vi "maze_v2.vi"   [LabVIEW 2012]
uses:
  <vilib>/NXT/Subs/MotorOutput.ctl
  <vilib>/NXT/Block Support/NXT_InputPort.ctl
  <vilib>/NXT/Dual Mode Library/Motors/MotorOn.vi
  <vilib>/NXT/Dual Mode Library/Motors/MotorReverse.vi
  <vilib>/NXT/Dual Mode Library/Motors/MotorBrake.vi
  <vilib>/NXT/Dual Mode Library/Display/clearDisplay.vi
  <vilib>/NXT/Dual Mode Library/Display/drawText.vi
  <vilib>/NXT/Dual Mode Library/Waits/Wait_Num(msec).vi
  <vilib>/NXT/Dual Mode Library/Display/drawLine.vi
  <vilib>/NXT/Dual Mode Library/Waits/Wait_Num.vi
  <vilib>/NXT/Dual Mode Library/Display/drawNumber.vi
types:
  T1 = typedef "MotorOutput.ctl" = u8
  T2 = typedef "LVHSConnector.ctl" = cluster{"Hardware":string, "Flattened String":string}
  T3 = typedef "NXT_InputPort.ctl" = u8
  T4 = cluster{"x":i32, "Start X":i16, "x":i32, "Start X":i16}
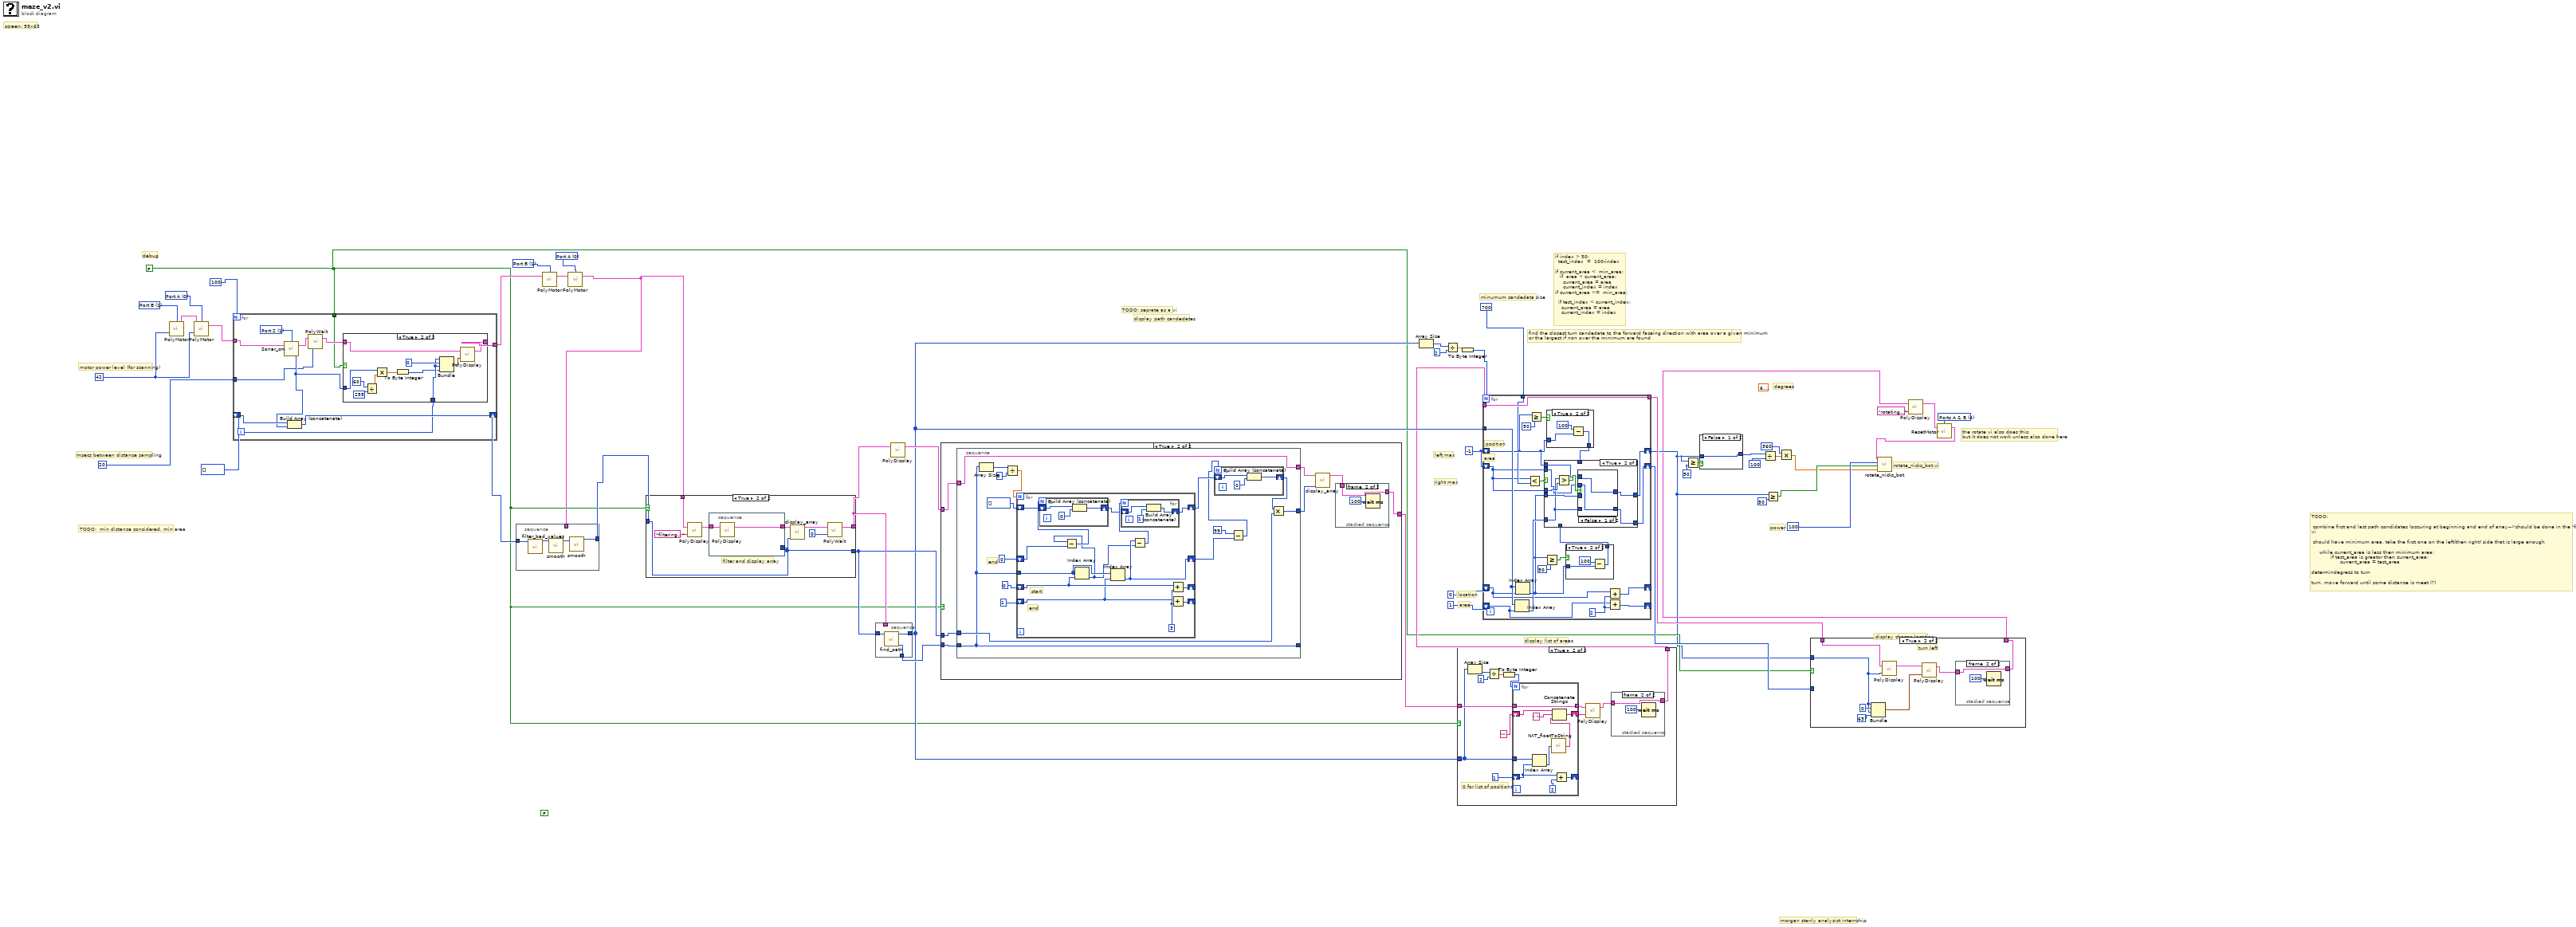
[diagram p0: block diagram]
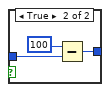
[diagram p2: hidden frame]
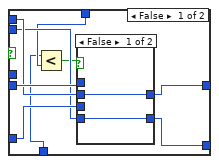
[diagram p8: hidden frame]
diagram:
  w5 = T1 4 items=["Port A"=0, "Port B"=1, "Port C"=2, "Ports A & B"=4, "Ports A & C"=5, "Ports B & C"=6, "All Ports"=3] ("Port (All Ports)")
  (unwired) 6.283185307179586 ("Pi Multiplied By 2")
  w21 = i16 -1 ("Start X")
  w38 = T1 0 items=["Port A"=0, "Port B"=1, "Port C"=2, "Ports A & B"=4, "Ports A & C"=5, "Ports B & C"=6, "as"=3] ("Output Port (All Ports)")
  w40 = T1 1 items=["Port A"=0, "Port B"=1, "Port C"=2, "Ports A & B"=4, "Ports A & C"=5, "Ports B & C"=6, "as"=3] ("Output Port (All Ports)")
  (unwired) FALSE
  w19 = FALSE
  w45 = 42 ("Power (75)")
  w47 = T1 0 items=["Port A"=0, "Port B"=1, "Port C"=2, "Ports A & B"=4, "Ports A & C"=5, "Ports B & C"=6, "as"=3] ("Output Port (All Ports)")
  w49 = T1 1 items=["Port A"=0, "Port B"=1, "Port C"=2, "Ports A & B"=4, "Ports A & C"=5, "Ports B & C"=6, "as"=3] ("Output Port (All Ports)")
  # "rotate_nicks_bot.vi"
  # "the rotate vi also does this,\nbut it does not work unless also done here"
  # "power"
  # "degrees"
  # "display chosen location"
  # "display list of areas"
  # "if index > 50;\n  test_index  =  100-index\n\nif current_area <  min_area:\n   if  area > current_area:\n     current_area = area\n     current_index = index\nif current_area >=  min_area:\n\n  if test_index < current_index:\n    current_area = area\n    current_index = index"
  # "morgan stanly analysist internship"
  # "minumum candedata size"
  # "find the closest turn candedate to the forward faceing direction with area over a given minimum\nor the largest if non over the minimum are found"
  # "TODO:  min distance considered, min area"
  # "msecs between distance sampling"
  # "motor power level (for scanning)"
  # "TODO: seprate as a vi"
  # "TODO:\n\n combine first and last path condidates (occuring at beginning and end of array-->should be done in the 'find paths' vi\n            \n should have minimum area, take the first one on the left(then right) side that is large enough\n\n     while current_area is less then minimum area:\n            if test_area is greator then current_area:\n                  current_area = test_area\n\ndetermindegress to turn\n\nturn, move forward until some distance is meet (?)"
  # "right max"
  # "left max"
  # "display path candedates"
  # "area"
  # "location"
  # "debug"
  # "screen: 99x63"
  n1 = call-poly <vilib>:"PolyMotor.vi"("Power (75)"=w45, "Output Port (All Ports)"=w49) -> ("NXT"=w48:T2)  [unwired: 2 in]
  n2 = call-poly <vilib>:"PolyMotor.vi"("Power (75)"=w45, "NXT"=w48, "Output Port (All Ports)"=w47) -> ("NXT"=w46:T2)  [unwired: 1 in]
  n3 = for {
    N: 100 -> [_]
    shift-right: [w57] -> w42
    shift-left: i16[] [] -> [w58]
    tunnel: w46 -> [w60]
    tunnel: [w54] -> w39
    tunnel: w19 -> [w53]
    tunnel: 20 -> [w50]
    i -> [w51]
    w59 = T3 1 items=["Port 1", "Port 2", "Port 3", "Port 4"] ("Port (Port 4)")
    n4 = call <vilib>:"Sonar_cm.vi"("NXT"=w60, "Port (Port 4)"=w59) -> ("Distance (cm)"=w52:i16, "NXT"=w56:T2)  [unwired: 1 in]
    n5 = Build Array (concatenate)(w58, w52) -> (w57:i16[])
    n6 = call-poly <vilib>:"PolyWait.vi"("Time (100 msec)"=w50, "NXT"=w56) -> ("NXT"=w55:T2)  [unwired: 2 in]
    n7 = case shown="True" w53 {
      tunnel: w55 -> [w61 w69]
      tunnel: [w61 w70] -> w54
      tunnel: w52 -> [_ w68]
      tunnel: w51 -> [_ w63]
      frame False {
      }
      frame True {
        n8 = Divide(x=i16 60 ("Start X"), y=i16 255 ("Start X")) -> (x/y=w66:dbl)
        n9 = Multiply(x=w68, y=w66) -> (x*y=w71:dbl)
        n10 = To Byte Integer(number=w71) -> (8bit integer=w62:i8)
        n11 = Bundle(w63, "Start X"=i16 0, w63, w62) -> (w64:cluster{i32, "Start X":i16, i32, i8})  [unwired: 1 in]
        n12 = call-poly <vilib>:"PolyDisplay.vi"("Line Parameters"=w64, "NXT"=w69) -> ("NXT"=w70:T2)  [unwired: 2 in]
      }
    }
  }
  n13 = call-poly <vilib>:"PolyMotor.vi"("NXT"=w39, "Port (All Ports)"=w40) -> ("NXT"=w41:T2)  [unwired: 2 in]
  n14 = call-poly <vilib>:"PolyMotor.vi"("NXT"=w41, "Port (All Ports)"=w38) -> ("NXT"=w1:T2)  [unwired: 2 in]
  n15 = stacked-sequence {
    tunnel: w42 -> [w74]
    tunnel: [w73] -> w37
    tunnel: w1 -> [_]
    frame #0 {
      n16 = call "filter_bad_values.vi"("Array 3"=w74) -> ("Array 4"=w75:i32[])  [unwired: 10 in]
      n17 = call "smooth.vi"("Array"=w75) -> ("Array 2"=w76:i32[])  [unwired: 10 in]
      n18 = call "smooth.vi"("Array"=w76) -> ("Array 2"=w73:i32[])  [unwired: 10 in]
    }
  }
  n19 = case shown="True" w19 {
    tunnel: w1 -> [w78 w83]
    tunnel: w37 -> [w77 w79]
    tunnel: [w78 w80] -> w34
    tunnel: [w77 w79] -> w36
    frame False {
    }
    frame True {
      # "filter and display array"
      n20 = call-poly <vilib>:"PolyDisplay.vi"("Text"="filtering...", "NXT"=w83) -> ("NXT"=w84:T2)  [unwired: 2 in]
      n21 = stacked-sequence {
        tunnel: [w88] -> w82
        tunnel: w79 -> [_]
        tunnel: w84 -> [w87]
        frame #0 {
          n22 = call-poly <vilib>:"PolyDisplay.vi"("NXT"=w87) -> ("NXT"=w88:T2)  [unwired: 3 in]
        }
      }
      n23 = call "display_array.vi"("array"=w79, "NXT"=w82) -> ("NXT 2"=w81:T2)  [unwired: 9 in]
      n24 = call-poly <vilib>:"PolyWait.vi"("Time (1 sec)"=i16 0 ("Start X"), "NXT"=w81) -> ("NXT"=w80:T2)  [unwired: 2 in]
    }
  }
  n25 = stacked-sequence {
    tunnel: w36 -> [w91]
    tunnel: [w90] -> w35
    tunnel: w34 -> [_]
    tunnel: [w89] -> w25
    frame #0 {
      n26 = call "find_path.vi"("Array"=w91) -> ("debug array"=w90:i32[], "Array 2"=w89:i32[])  [unwired: 9 in]
    }
  }
  n27 = call-poly <vilib>:"PolyDisplay.vi"("NXT"=w34) -> ("NXT"=w33:T2)  [unwired: 3 in]
  n28 = case shown="True" w19 {
    tunnel: w35 -> [_ w98]
    tunnel: w33 -> [w92 w97]
    tunnel: [w92 w94] -> w27
    tunnel: w36 -> [_ w99]
    frame False {
    }
    frame True {
      n29 = stacked-sequence {
        tunnel: w99 -> [w113]
        tunnel: [w112] -> w93
        tunnel: w98 -> [w102]
        tunnel: w97 -> [w103]
        tunnel: [w103] -> w96
        tunnel: [w102] -> _
        frame #0 {
          # "end"
          n30 = Array Size(array=w102) -> (size(s)=w106:i32)
          n31 = Divide(x=w106, y=3) -> (x/y=w104:dbl)
          n32 = for {
            N: w104 -> [_]
            shift-right: [w133] -> _
            shift-left: i16 0 ("Start X") -> [w130]
            shift-right: [w132] -> _
            shift-left: i16 1 ("Start X") -> [w129]
            shift-right: [w121] -> w111
            shift-left: i16[] [] -> [w123]
            tunnel: w102 -> [w128]
            shift-right: [w126] -> w108
            shift-left: i16 0 ("Start X") -> [w127]
            w134 = 3 ("y")
            # "end"
            # "start"
            n33 = Index Array(array=w128, index=w130) -> (element=w125:i32)
            n34 = Subtract(x=w125, y=w127) -> (x-y=w131:i32)
            n35 = for {
              N: w131 -> [_]
              shift-right: [w139] -> w122
              shift-left: w123 -> [w140]
              n36 = Build Array (concatenate)(w140, i16 0 ("Start X")) -> (w139:i16[])
            }
            n37 = Index Array(array=w128, index=w129) -> (element=w126:i32)
            n38 = Subtract(x=w126, y=w125) -> (x-y=w124:i32)
            n39 = for {
              N: w124 -> [_]
              shift-right: [w135] -> w121
              shift-left: w122 -> [w136]
              n40 = Build Array (concatenate)(w136, i16 1 ("Start X")) -> (w135:i16[])
            }
            n41 = Add(x=w130, y=w134) -> (x+y=w133:i32)
            n42 = Add(x=w129, y=w134) -> (x+y=w132:i32)
          }
          n43 = Subtract(x=i16 99 ("Start X"), y=w108) -> (x-y=w107:i32)
          n44 = for {
            N: w107 -> [_]
            shift-right: [w119] -> w110
            shift-left: w111 -> [w120]
            n45 = Build Array (concatenate)(w120, i16 0 ("Start X")) -> (w119:i16[])
          }
          n46 = Multiply(x=w110, y=w113) -> (x*y=w112:i32[])
        }
      }
      n47 = call "display_array.vi"("array"=w93, "NXT"=w96) -> ("NXT 2"=w95:T2)  [unwired: 9 in]
      n48 = stacked-sequence {
        tunnel: [_ w100] -> w94
        tunnel: w95 -> [_ w100]
        frame #0 {
        }
        frame #1 {
          n49 = Wait (ms)(milliseconds to wait=u32 100) -> ()  [unwired: 1 out]
        }
      }
    }
  }
  n50 = Array Size(array=w25) -> (size(s)=w30:i32)
  n51 = Divide(x=w30, y=2) -> (x/y=w28:dbl)
  n52 = case shown="True" w19 {
    tunnel: w27 -> [w141 w150]
    tunnel: w25 -> [_ w144]
    tunnel: [w141 w143] -> w24
    frame False {
    }
    frame True {
      # "0 for list of positions"
      n53 = Array Size(array=w144) -> (size(s)=w148:i32)
      n54 = Divide(x=w148, y=2) -> (x/y=w146:dbl)
      n55 = To Byte Integer(number=w146) -> (8bit integer=w145:i8)
      n56 = for {
        N: w145 -> [_]
        tunnel: w150 -> [w162]
        tunnel: [w162] -> w152
        shift-right: [w163] -> w151
        shift-left: "" ("Text") -> [w165]
        shift-right: [w160] -> _
        shift-left: i16 1 ("Start X") -> [w158]
        tunnel: w144 -> [w157]
        n57 = Index Array(array=w157, index=w158) -> (element=w156:i32)
        n58 = call <vilib>:"NXT_floatToString.vi"("number"=w156) -> ("string"=w164:string)
        n59 = Concatenate Strings(w165, " " ("Text"), w164) -> (w163:string)
        n60 = Add(x=w158, y=i16 2 ("Start X")) -> (x+y=w160:i16)
      }
      n61 = call-poly <vilib>:"PolyDisplay.vi"("Text"=w151, "NXT"=w152) -> ("NXT"=w142:T2)  [unwired: 2 in]
      n62 = stacked-sequence {
        tunnel: w142 -> [_ w154]
        tunnel: [_ w154] -> w143
        frame #0 {
        }
        frame #1 {
          n63 = Wait (ms)(milliseconds to wait=u32 100) -> ()  [unwired: 1 out]
        }
      }
    }
  }
  n64 = To Byte Integer(number=w28) -> (8bit integer=w26:i8)
  n65 = for {
    N: w26 -> [_]
    tunnel: w25 -> [w186]
    shift-right: [w185] -> _
    shift-left: i16 0 ("Start X") -> [w166]
    shift-right: [w184] -> _
    shift-left: i16 1 ("Start X") -> [w182]
    shift-right: [w176] -> w9
    shift-left: w21 -> [w170]
    shift-right: [w175] -> w20
    shift-left: w21 -> [w167]
    tunnel: w24 -> [w181]
    tunnel: i16 700 ("Start X") -> [w168]
    tunnel: [w181] -> w14
    w183 = i16 2 ("Start X")
    # "area"
    # "position"
    n66 = Index Array(array=w186, index=w182) -> (element=w177:i32)
    n67 = Index Array(array=w186, index=w166) -> (element=w169:i32)
    n68 = Less?(x=w167, y=w168) -> (x < y?=w178:bool)
    n69 = Greater Or Equal?(x=w170, y=i16 50 ("Start X")) -> (x >= y?=w179:bool)
    n70 = Greater Or Equal?(x=w169, y=i16 50 ("Start X")) -> (x >= y?=w173:bool)
    n71 = case shown="True" w179 {
      tunnel: w170 -> [w216 w217]
      tunnel: [w216 w219] -> w174
      frame False {
      }
      frame True {
        n72 = Subtract(x=i16 100 ("Start X"), y=w217) -> (x-y=w219:i32)
      }
    }
    n73 = case shown="True" w173 {
      tunnel: w169 -> [w187 w189]
      tunnel: [w187 w188] -> w171
      frame False {
      }
      frame True {
        n74 = Subtract(x=i16 100 ("Start X"), y=w189) -> (x-y=w188:i32)
      }
    }
    n75 = case shown="True" w178 {
      tunnel: w169 -> [w199 w209]
      tunnel: w177 -> [w198 w207]
      tunnel: [w197 w208] -> w176
      tunnel: [w196 w206] -> w175
      tunnel: w174 -> [w193 _]
      tunnel: w171 -> [w192 _]
      tunnel: w170 -> [w195 w205]
      tunnel: w167 -> [w194 w204]
      tunnel: w167 -> [_ w211]
      frame False {
        n76 = Less?(x=w192, y=w193) -> (x < y?=w191:bool)
        n77 = case shown="False" w191 {
          tunnel: w199 -> [_ w203]
          tunnel: w198 -> [_ w202]
          tunnel: [w201 w203] -> w197
          tunnel: [w200 w202] -> w196
          tunnel: w195 -> [w201 _]
          tunnel: w194 -> [w200 _]
          frame False {
          }
          frame True {
          }
        }
      }
      frame True {
        n78 = Greater?(x=w207, y=w211) -> (0:w210:bool)
        n79 = case shown="False" w210 {
          tunnel: w209 -> [_ w215]
          tunnel: [w212 w215] -> w208
          tunnel: w207 -> [_ w214]
          tunnel: [w213 w214] -> w206
          tunnel: w205 -> [w212 _]
          tunnel: w204 -> [w213 _]
          frame False {
          }
          frame True {
          }
        }
      }
    }
    n80 = Add(x=w166, y=w183) -> (x+y=w185:i16)
    n81 = Add(x=w182, y=w183) -> (x+y=w184:i16)
  }
  n82 = Greater Or Equal?(x=w9, y=i16 50 ("Start X")) -> (x >= y?=w11:bool)
  n83 = case shown="False" w11 {
    tunnel: w9 -> [w220 w221]
    tunnel: [w220 w223] -> w10
    frame False {
    }
    frame True {
      n84 = Subtract(x=i16 100 ("Start X"), y=w221) -> (x-y=w223:i32)
    }
  }
  n85 = Divide(x=w10, y=i16 100 ("Start X")) -> (x/y=w16:dbl)
  n86 = Greater Or Equal?(x=w9, y=i16 50 ("Start X")) -> (x >= y?=w8:bool)
  n87 = Multiply(x=i16 360 ("Start X"), y=w16) -> (x*y=w2:dbl)
  n88 = case shown="True" w19 {
    tunnel: w9 -> [_ w227]
    tunnel: w14 -> [w224 w229]
    tunnel: [w224 w225] -> w7
    tunnel: w20 -> [_ _]
    frame False {
      # "turn right"
    }
    frame True {
      # "turn left"
      n89 = Bundle("x"=w227, "Start X"=i16 0, "x"=w227, "Start X"=i16 63) -> (w228:T4)  [unwired: 1 in]
      n90 = call-poly <vilib>:"PolyDisplay.vi"("number"=w227, "NXT"=w229) -> ("NXT"=w232:T2)  [unwired: 2 in]
      n91 = call-poly <vilib>:"PolyDisplay.vi"("Line Parameters"=w228, "NXT"=w232) -> ("NXT"=w226:T2)  [unwired: 2 in]
      n92 = stacked-sequence {
        tunnel: w226 -> [_ w233]
        tunnel: [_ w233] -> w225
        frame #0 {
        }
        frame #1 {
          n93 = Wait (ms)(milliseconds to wait=u32 100) -> ()  [unwired: 1 out]
        }
      }
    }
  }
  n94 = call-poly <vilib>:"PolyDisplay.vi"("Text"="rotating...", "NXT"=w7) -> ("NXT"=w4:T2)  [unwired: 2 in]
  n95 = call <vilib>:"ResetMotor.vi"("NXT"=w4, "Port (All Ports)"=w5) -> ("NXT"=w3:T2)  [unwired: 2 in]
  n96 = call "rotate_nicks_bot.vi"("degrees to  rotate"=w2, "right(T)/left(F)"=w8, "power"=u16 100 ("Max Value"), "NXT 2"=w3) -> ()  [unwired: 7 in, 1 out]
